vi "Add List Image Border.vi"(9 "Background Color":u32(colorbox)=16777215, 11 "new picture in":picture) -> (3 "new picture out":picture)   [LabVIEW 2016, in "MetaDataObj.lvclass"]
uses:
  <resource>/dialog/NewProjectWizard/MetaDataObj/MetaDataObj.lvclass
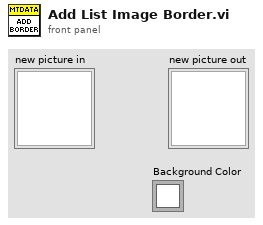
[diagram p1: front panel]
types:
  T1 = typedef "imagedata.ctl" = cluster{"image type":i32, "image depth":i32, "image":u8[], "mask":u8[], "colors":u32[], "Rectangle":cluster{"left":i16, "top":i16, "right":i16, "bottom":i16}}
  T2 = cluster{"left":i16, "top":i16, "right":i16, "bottom":i16}
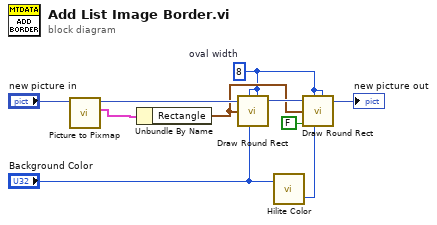
[diagram p0: block diagram]
diagram:
  w1 = i16 8  # oval width
  n1 = call <vilib>:"Picture to Pixmap.vi"("picture"="new picture in") -> ("image data"=w6:T1, "new picture"=w7:picture)  [unwired: 9 in]
  n2 = Unbundle By Name(w6) -> ("Rectangle"=w2:T2)
  n3 = call <vilib>:"Draw Round Rect.vi"("picture"=w7, "oval width"=w1, "rect"=w2, "color(black)"="Background Color", "oval height"=w1) -> ("new picture"=w4:picture)  [unwired: 4 in]
  n4 = call <vilib>:"Hilite Color.vi"("Color In"="Background Color") -> ("Shadow"=w3:u32)  [unwired: 1 in, 1 out]
  n5 = call <vilib>:"Draw Round Rect.vi"("picture"=w4, "oval width"=w1, "rect"=w2, "fill?(F)"=FALSE, "color(black)"=w3, "oval height"=w1) -> ("new picture"=→"new picture out":picture)  [unwired: 3 in]
